vi "Rinocloud_HTTP_upload_file.vi"(4 "Store locally":bool=TRUE, 5 "Extra metadata array":T2(array[cluster])=[{"Attribute"="", "Value"="", "Data type"=enum."<null>"}, {"Attribute"="Amplitude", "Value"="10", "Data type"=enum."<null>"}], 6 "Path in":path, 7 "Parent ID":string, 8 "error in (no error)":errorcluster, 9 "Notes":string, 10 "Tags":string, 11 "Name":string) -> (0 "error out":errorcluster, 2 "Path out":path, 3 "Status":T1={"headers"="", "body"="", "ID"="", "Saved"=TRUE})   [LabVIEW 2013, in "Rinocloud Library.lvlib"]
uses:
  Rinocloud Library.lvlib
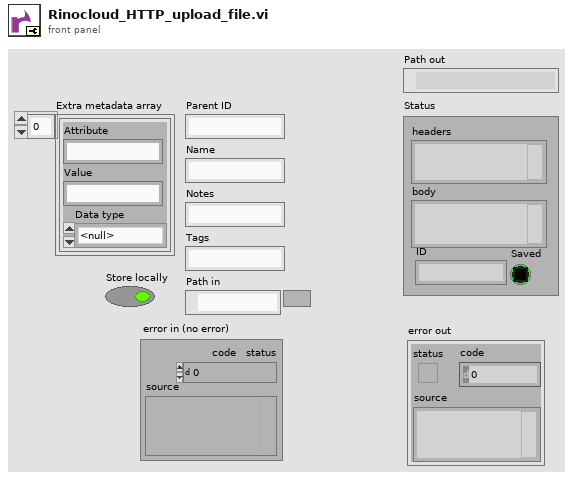
[diagram p1: front panel]
types:
  T1 = cluster{"headers":string, "body":string, "ID":string, "Saved":bool}
  T2 = cluster{"Attribute":string, "Value":string, "Data type":enum16{"Numeric", "String", "1D array of strings", "1D array of doubles", "Data JSON string", "<null>"}}[]
  T3 = cluster{"Name":string, "Notes":string, "Tags":string}
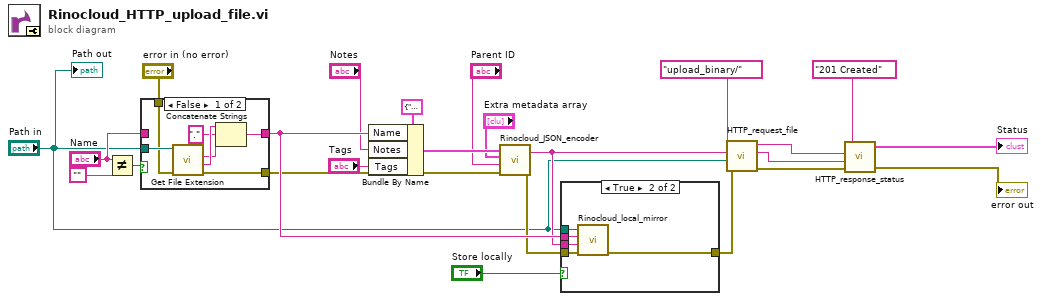
[diagram p0: block diagram]
diagram:
  n1 = Not Equal?(x="Name", y="") -> (x != y?=w14:bool)
  n2 = case shown="False" w14 {
    tunnel: [w30 w33] -> w19
    tunnel: "Name" -> [_ w33]
    tunnel: "Path in" -> [w31 _]
    tunnel: "error in (no error)" -> [w26 w32]
    tunnel: [w25 w32] -> w17
    frame False {
      n3 = call <vilib>:"Get File Extension.vi"("error in (no error)"=w26, "file"=w31) -> ("error out"=w25:errorcluster, "filename without extension"=w29:string, "lowercase file extension"=w27:string)  [unwired: 6 in, 1 out]
      n4 = Concatenate Strings(w29, "." ("string"), w27) -> (w30:string)
    }
    frame True {
    }
  }
  n5 = Bundle By Name(cluster=T3 {"Name"="", "Notes"="", "Tags"=""} ("Metadata"), "Name"=w19, "Notes"="Notes", "Tags"="Tags") -> (w10:T3)
  n6 = call "Rinocloud_JSON_encoder.vi"("Metadata"=w10, "Extra metadata array"="Extra metadata array", "parent ID"="Parent ID", "error in (no error)"=w17) -> ("JSON payload"=w5:string, "error out"=w18:errorcluster)  [unwired: 1 in]
  n7 = case shown="True" "Store locally" {
    tunnel: w19 -> [_ w39]
    tunnel: w18 -> [w34 w38]
    tunnel: [w34 w37] -> w6
    tunnel: w5 -> [_ w36]
    tunnel: "Path in" -> [_ w35]
    frame False {
    }
    frame True {
      n8 = call "Rinocloud_local_mirror.vi"("error in"=w38, "JSON payload"=w36, "file name"=w39, "file path"=w35) -> ("error out"=w37:errorcluster)  [unwired: 7 in]
    }
  }
  n9 = call "HTTP_request_file.vi"("error in (no error)"=w6, "Path"="Path in", "JSON payload"=w5, "Endpoint"="upload_binary/") -> ("error out"=w22:errorcluster, "Body"=w24:string, "Headers"=w23:string)  [unwired: 1 in]
  n10 = call "HTTP_response_status.vi"("error in (no error)"=w22, "body"=w24, "headers"=w23, "HTTP status"="201 Created") -> ("error out"=→"error out":errorcluster, "Status"=→"Status":T1)  [unwired: 1 in]
  "Path out" <- "Path in"
